vi "Input.vi"(7 "Actor in":refnum<class "Actor.lvclass">, 8 "Error in":errorcluster, 10 "Msg DVR in":refnum<data-value>) -> (0 "Error out":errorcluster, 2 "Msg DVR out":refnum<data-value>, 5 "Actor out":refnum<class "Actor.lvclass">)   [LabVIEW 2020, in "_Template.lvlib" / "Templates.lvlib" / "TEMPLATE jettl Msg.lvlib" / "TEMPLATE Msg Input.lvclass"]
uses:
  TEMPLATE Msg Input.lvclass
  TEMPLATE Msg Input.lvclass/TEMPLATE Msg Input.ctl
  TEMPLATE jettl Msg/TEMPLATE jettl Msg.lvclass
  jettl/jettl/Actor/Actor.lvclass
  jettl/jettl/Unified Actor Relation.ctl
  jettl/jettl/jettl.lvlib
  jettl/jettl/Teller.ctl
  jettl/jettl/Msg Input/Msg Input.lvclass
  jettl/jettl/Msg.ctl
  jettl/jettl/Msg Output/Msg Output.lvclass
  jettl/jettl/Msg/Msg.lvclass
panel:
  # "This front panel should not be manipulated."
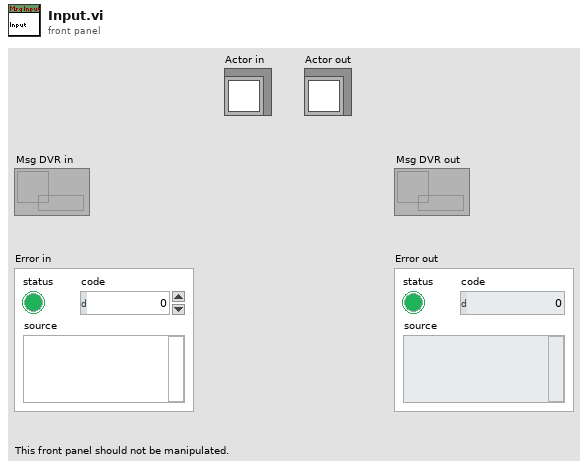
[diagram p1: front panel]
types:
  T1 = typedef "jettl.lvlib/Msg.ctl" = cluster{"Msg":refnum<class "Msg.lvclass">, "Msg Input":refnum<class "Msg Input.lvclass">, "Msg Output":refnum<class "Msg Output.lvclass">, "Teller":T2}
  T2 = typedef "jettl.lvlib/Teller.ctl" = cluster{"Unified Actor Alias":string, "Unified Actor Relation":T3, "Absolute Time":timestamp, "Relative Time":dbl, "Msg DVR UID":i32}
  T3 = typedef "jettl.lvlib/Unified Actor Relation.ctl" = enum16{"Self", "Parent", "Child"}
  T4 = typedef "_Template.lvlib/Templates.lvlib/TEMPLATE jettl Msg.lvlib/Input.ctl" = cluster{"Placeholder":bool}
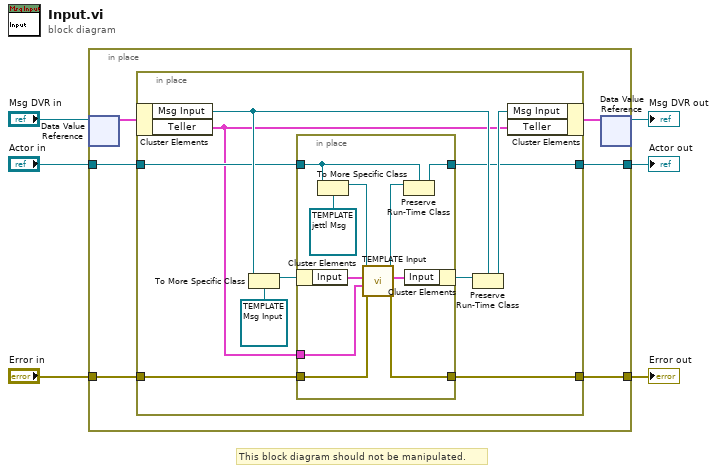
[diagram p0: block diagram]
diagram:
  # "This block diagram should not be manipulated."
  n1 = in-place {
    in-place-border: "Error in" -> [w12]
    in-place-border: [w11] -> w5
    in-place-border: "Actor in" -> [w10]
    in-place-border: [w9] -> w3
    n2 = in-place-dvr #1("Msg DVR in") -> (w8:T1)  [unwired: 1 out]
    n3 = in-place {
      in-place-border: w12 -> [w22]
      in-place-border: [w21] -> w11
      in-place-border: w10 -> [w15]
      in-place-border: [w14] -> w9
      n4 = in-place-cluster #2(w8) -> ("Msg Input"=w18:refnum<class "Msg Input.lvclass">, "Teller"=w13:T2)
      n5 = To More Specific Class(target class=refnum<class "TEMPLATE Msg Input.lvclass"> refnum ("_Template.lvlib:Templates.lvlib:TEMPLATE jettl Msg.lvlib:TEMPLATE Msg Input.lvlib:TEMPLATE Msg Input.lvclass"), reference=w18) -> (specific class reference=w19:refnum<class "TEMPLATE Msg Input.lvclass">)  [unwired: 1 in, 1 out]
      n6 = in-place {
        in-place-border: w22 -> [w32]
        in-place-border: [w31] -> w21
        in-place-border: w15 -> [w26]
        in-place-border: [w27] -> w14
        in-place-border: w13 -> [w23]
        n7 = in-place-cluster #3(w19) -> ("Input"=w30:T4)
        n8 = To More Specific Class(target class=refnum<class "TEMPLATE jettl Msg.lvclass"> refnum ("_Template.lvlib:Templates.lvlib:TEMPLATE jettl Msg.lvlib:TEMPLATE jettl Msg.lvclass"), reference=w26) -> (specific class reference=w28:refnum<class "TEMPLATE jettl Msg.lvclass">)  [unwired: 1 in, 1 out]
        n9 = call-dynamic "TEMPLATE Input.vi"("Error in"=w32, "Teller"=w23, "Input in"=w30, "TEMPLATE jettl Msg in"=w28) -> ("Error out"=w31:errorcluster, "Input out"=w24:T4, "TEMPLATE jettl Msg out"=w25:refnum<class "TEMPLATE jettl Msg.lvclass">)  [unwired: 5 in]
        n10 = Preserve Run-Time Class(object in=w25, 2:w26) -> (object out=w27:refnum<class "Actor.lvclass">)  [unwired: 1 in, 1 out]
        n11 = in-place-cluster #3("Input"=w24) -> (w17:refnum<class "TEMPLATE Msg Input.lvclass">)
      }
      n12 = Preserve Run-Time Class(object in=w17, 2:w18) -> (object out=w16:refnum<class "Msg Input.lvclass">)  [unwired: 1 in, 1 out]
      n13 = in-place-cluster #2("Msg Input"=w16, "Teller"=w13) -> (w7:T1)
    }
    n14 = in-place-dvr #1(w7) -> (→"Msg DVR out":refnum<data-value>)  [unwired: 1 out]
  }
  "Actor out" <- w3
  "Error out" <- w5
